vi "Updata Monitor setting.vi"(7 "Channel number":i32=4, 8 "XY Graph REF":refnum<vi>, 9 "new plot setting":T1(array[cluster]), 10 "old plot setting":T1(array[cluster]), 11 "plot setting REF":refnum<vi>) -> ()   [LabVIEW 2023]
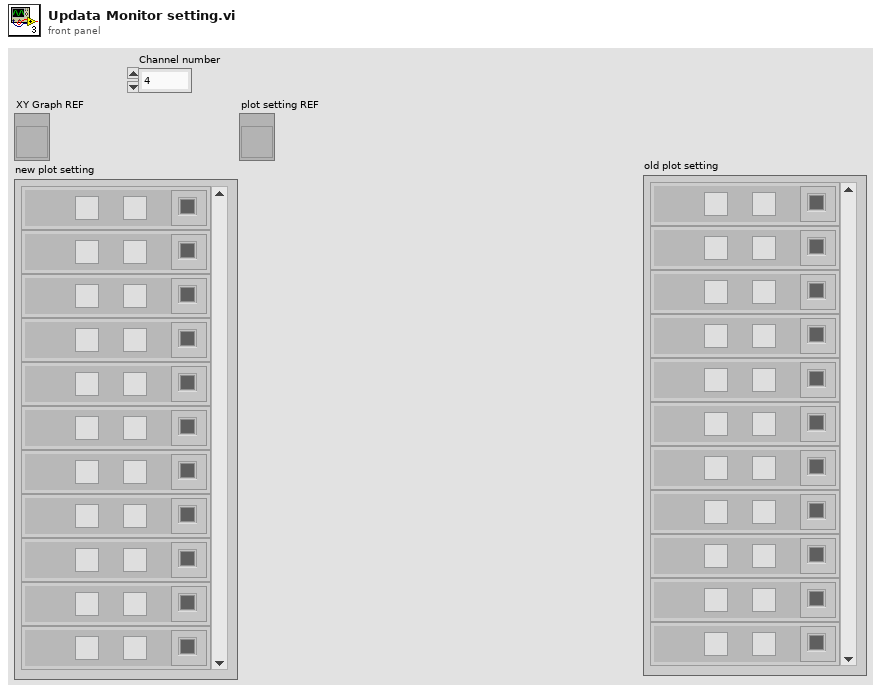
[diagram p1: front panel]
types:
  T1 = cluster{"V plot":bool, "I plot":bool, "Plot colour":u32, "Channel name\n":string}[]
  T2 = cluster{"V plot":bool, bool, "Plot colour":u32, "Channel name\n":string}
  T3 = cluster{bool, "I plot":bool, "Plot colour":u32, "Channel name\n":string}
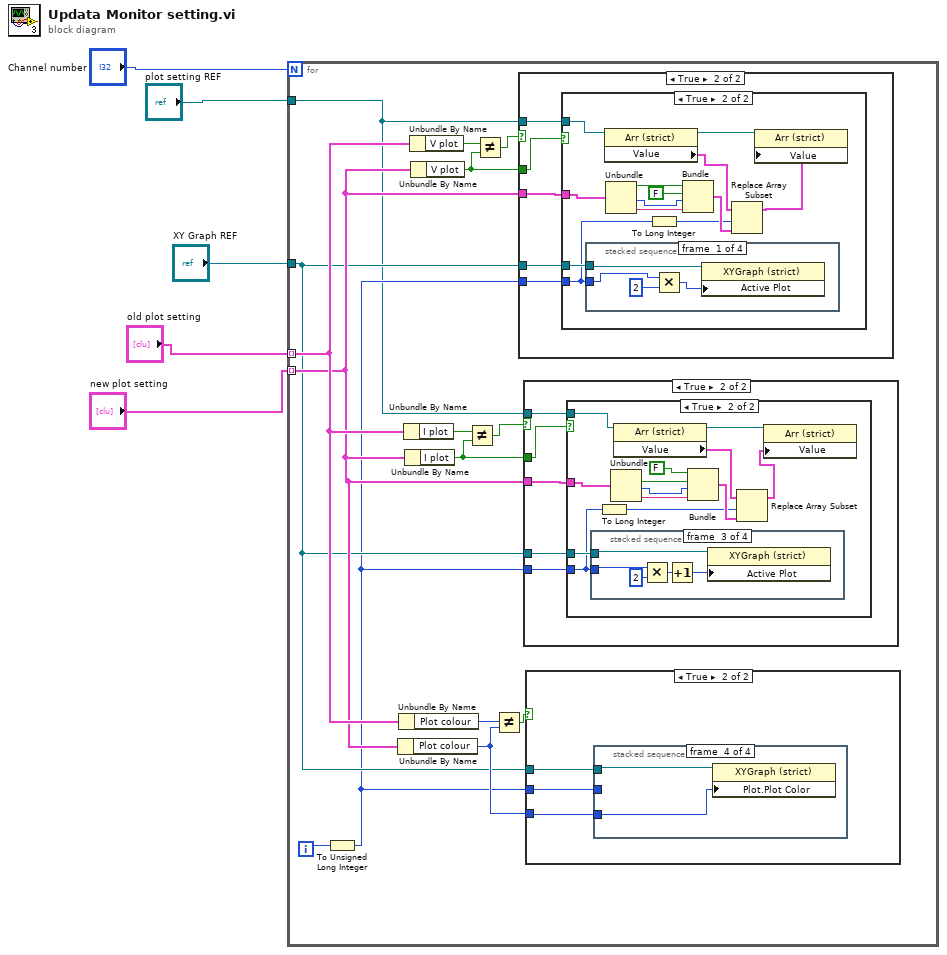
[diagram p0: block diagram]
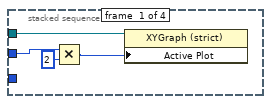
[diagram p3: hidden frame]
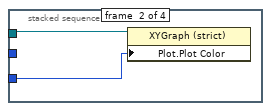
[diagram p4: hidden frame]
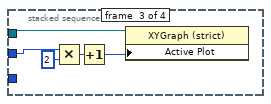
[diagram p5: hidden frame]
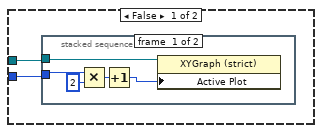
[diagram p7: hidden frame]
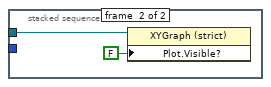
[diagram p8: hidden frame]
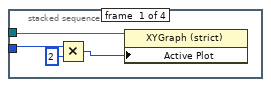
[diagram p9: hidden frame]
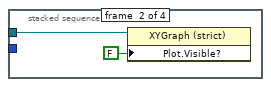
[diagram p10: hidden frame]
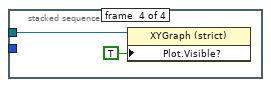
[diagram p11: hidden frame]
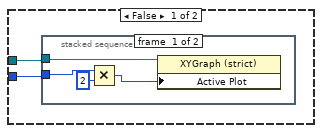
[diagram p13: hidden frame]
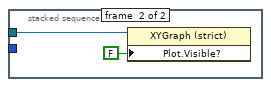
[diagram p14: hidden frame]
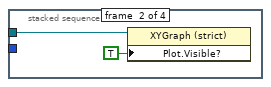
[diagram p15: hidden frame]
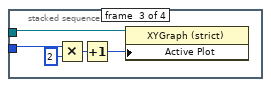
[diagram p16: hidden frame]
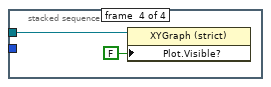
[diagram p17: hidden frame]
diagram:
  n1 = for {
    N: "Channel number" -> [_]
    tunnel: "XY Graph REF" -> [w8]
    tunnel: "old plot setting" -> [w10] mode=indexing
    tunnel: "new plot setting" -> [w9] mode=indexing
    tunnel: "plot setting REF" -> [w6]
    i -> [w17]
    n2 = To Unsigned Long Integer(number=w17) -> (unsigned 32bit integer=w7:u32)
    n3 = Unbundle By Name(w9) -> ("Plot colour"=w12:u32)
    n4 = Unbundle By Name(w10) -> ("Plot colour"=w13:u32)
    n5 = Unbundle By Name(w10) -> ("I plot"=w16:bool)
    n6 = Unbundle By Name(w9) -> ("I plot"=w14:bool)
    n7 = Unbundle By Name(w10) -> ("V plot"=w20:bool)
    n8 = Unbundle By Name(w9) -> ("V plot"=w18:bool)
    n9 = Not Equal?(x=w16, y=w14) -> (x != y?=w15:bool)
    n10 = Not Equal?(x=w20, y=w18) -> (x != y?=w19:bool)
    n11 = Not Equal?(x=w13, y=w12) -> (x != y?=w11:bool)
    n12 = case shown="True" w19 {
      tunnel: w18 -> [_ w81]
      tunnel: w9 -> [_ w80]
      tunnel: w8 -> [_ w79]
      tunnel: w7 -> [_ w78]
      tunnel: w6 -> [_ w77]
      frame False {
      }
      frame True {
        n13 = case shown="True" w81 {
          tunnel: w80 -> [_ w102]
          tunnel: w79 -> [w83 w96]
          tunnel: w78 -> [w82 w95]
          tunnel: w77 -> [_ w91]
          frame False {
            n14 = stacked-sequence {
              tunnel: w83 -> [w87 w89]
              tunnel: w82 -> [w84 _]
              frame #0 {
                n15 = Multiply(x=w84, y=u32 2) -> (x*y=w85:u32)
                n16 = property class="XYGraph (strict)"(reference=w87, "Active Plot"=w85) -> ()  [unwired: 1 in, 2 out]
              }
              frame #1 {
                n17 = property class="XYGraph (strict)"(reference=w89, "Plot.Visible?"=FALSE ("Plot.Visible")) -> ()  [unwired: 1 in, 2 out]
              }
            }
          }
          frame True {
            n18 = stacked-sequence {
              tunnel: w96 -> [w106 w108 w113 w115]
              tunnel: w95 -> [w104 _ w109 _]
              frame #0 {
                n19 = Multiply(x=w104, y=u32 2) -> (x*y=w103:u32)
                n20 = property class="XYGraph (strict)"(reference=w106, "Active Plot"=w103) -> ()  [unwired: 1 in, 2 out]
              }
              frame #1 {
                n21 = property class="XYGraph (strict)"(reference=w108, "Plot.Visible?"=TRUE ("Plot.Visible")) -> ()  [unwired: 1 in, 2 out]
              }
              frame #2 {
                n22 = Multiply(x=w109, y=u32 2) -> (x*y=w111:u32)
                n23 = Increment(x=w111) -> (x+1=w110:u32)
                n24 = property class="XYGraph (strict)"(reference=w113, "Active Plot"=w110) -> ()  [unwired: 1 in, 2 out]
              }
              frame #3 {
                n25 = property class="XYGraph (strict)"(reference=w115, "Plot.Visible?"=FALSE ("Plot.Visible")) -> ()  [unwired: 1 in, 2 out]
              }
            }
            n26 = property class="Arr (strict)"(reference=w91) -> (reference out=w90:refnum<vi>, "Value"=w93:T1)  [unwired: 1 in, 1 out]
            n27 = Unbundle(w102) -> ("V plot"=w101:bool, "Plot colour"=w98:u32, "Channel name"=w99:string)  [unwired: 1 out]
            n28 = To Long Integer(number=w95) -> (32bit integer=w94:i32)
            n29 = Bundle("V plot"=w101, FALSE, "Plot colour"=w98, "Channel name"=w99) -> (w97:T2)  [unwired: 1 in]
            n30 = Replace Array Subset(array=w93, new element=w97, index=w94) -> (w92:T1)
            n31 = property class="Arr (strict)"(reference=w90, "Value"=w92) -> ()  [unwired: 1 in, 2 out]
          }
        }
      }
    }
    n32 = case shown="True" w15 {
      tunnel: w14 -> [_ w41]
      tunnel: w9 -> [_ w40]
      tunnel: w8 -> [_ w39]
      tunnel: w7 -> [_ w38]
      tunnel: w6 -> [_ w37]
      frame False {
      }
      frame True {
        n33 = case shown="True" w41 {
          tunnel: w40 -> [_ w63]
          tunnel: w39 -> [w43 w59]
          tunnel: w38 -> [w42 w56]
          tunnel: w37 -> [_ w54]
          frame False {
            n34 = stacked-sequence {
              tunnel: w43 -> [w48 w50]
              tunnel: w42 -> [w44 _]
              frame #0 {
                n35 = Multiply(x=w44, y=u32 2) -> (x*y=w46:u32)
                n36 = Increment(x=w46) -> (x+1=w45:u32)
                n37 = property class="XYGraph (strict)"(reference=w48, "Active Plot"=w45) -> ()  [unwired: 1 in, 2 out]
              }
              frame #1 {
                n38 = property class="XYGraph (strict)"(reference=w50, "Plot.Visible?"=FALSE ("Plot.Visible")) -> ()  [unwired: 1 in, 2 out]
              }
            }
          }
          frame True {
            n39 = stacked-sequence {
              tunnel: w59 -> [w67 w69 w74 w76]
              tunnel: w56 -> [w64 _ w70 _]
              frame #0 {
                n40 = Multiply(x=w64, y=u32 2) -> (x*y=w65:u32)
                n41 = property class="XYGraph (strict)"(reference=w67, "Active Plot"=w65) -> ()  [unwired: 1 in, 2 out]
              }
              frame #1 {
                n42 = property class="XYGraph (strict)"(reference=w69, "Plot.Visible?"=FALSE ("Plot.Visible")) -> ()  [unwired: 1 in, 2 out]
              }
              frame #2 {
                n43 = Multiply(x=w70, y=u32 2) -> (x*y=w72:u32)
                n44 = Increment(x=w72) -> (x+1=w71:u32)
                n45 = property class="XYGraph (strict)"(reference=w74, "Active Plot"=w71) -> ()  [unwired: 1 in, 2 out]
              }
              frame #3 {
                n46 = property class="XYGraph (strict)"(reference=w76, "Plot.Visible?"=TRUE ("Plot.Visible")) -> ()  [unwired: 1 in, 2 out]
              }
            }
            n47 = To Long Integer(number=w56) -> (32bit integer=w55:i32)
            n48 = Unbundle(w63) -> ("I plot"=w57:bool, "Plot colour"=w61:u32, "Channel name"=w62:string)  [unwired: 1 out]
            n49 = property class="Arr (strict)"(reference=w54) -> (reference out=w53:refnum<vi>, "Value"=w52:T1)  [unwired: 1 in, 1 out]
            n50 = Bundle(FALSE, "I plot"=w57, "Plot colour"=w61, "Channel name"=w62) -> (w60:T3)  [unwired: 1 in]
            n51 = Replace Array Subset(array=w52, new element=w60, index=w55) -> (w51:T1)
            n52 = property class="Arr (strict)"(reference=w53, "Value"=w51) -> ()  [unwired: 1 in, 2 out]
          }
        }
      }
    }
    n53 = case shown="True" w11 {
      tunnel: w12 -> [_ w21]
      tunnel: w8 -> [_ w23]
      tunnel: w7 -> [_ w22]
      frame False {
      }
      frame True {
        n54 = stacked-sequence {
          tunnel: w23 -> [w27 w28 w34 w35]
          tunnel: w22 -> [w25 _ w31 _]
          tunnel: w21 -> [_ w29 _ w36]
          frame #0 {
            n55 = Multiply(x=w25, y=u32 2) -> (x*y=w24:u32)
            n56 = property class="XYGraph (strict)"(reference=w27, "Active Plot"=w24) -> ()  [unwired: 1 in, 2 out]
          }
          frame #1 {
            n57 = property class="XYGraph (strict)"(reference=w28, "Plot.Plot Color"=w29) -> ()  [unwired: 1 in, 2 out]
          }
          frame #2 {
            n58 = Multiply(x=w31, y=u32 2) -> (x*y=w32:u32)
            n59 = Increment(x=w32) -> (x+1=w30:u32)
            n60 = property class="XYGraph (strict)"(reference=w34, "Active Plot"=w30) -> ()  [unwired: 1 in, 2 out]
          }
          frame #3 {
            n61 = property class="XYGraph (strict)"(reference=w35, "Plot.Plot Color"=w36) -> ()  [unwired: 1 in, 2 out]
          }
        }
      }
    }
  }
